vi "Test DMM-Readout.vi"() -> ()   [LabVIEW 2015, in "CS++DMM.lvlib"]
uses:
  CS++DMM.lvlib
  CSPP_Core/Classes/CS++BaseClasses/Factory/CS++Factory.lvclass
  CSPP_Core/Classes/CS++BaseClasses/Factory/CS++Factory.lvclass/CS++Factory.ctl
  CS++DMM.lvclass
  CSPP_Core/Actors/CS++DeviceActor/CS++DeviceActor.lvclass/CS++DeviceActor.ctl
  CSPP_Core/Actors/CS++DeviceActor/Read Resource Name.vi
  CSPP_Core/Actors/CS++DeviceActor/CS++DeviceActor.lvclass
  CSPP_Core/Actors/CS++BaseActor/CS++BaseActor.lvclass
panel:
  in  "CS++Object Names":string[](array[string])=["DMM3458A-GPIB0-21", "DMM3458A-GPIB0-22"]
  out "Last Time":timestamp format="%<%H:%M:%S%1u>T"
  in  "File Path Control":path=path "C:/User/Brand/LVP/STF/STF.ini"
  out "error out":errorcluster
  in  "Stop Button":bool
  out "Readings":dbl[](array[numeric])
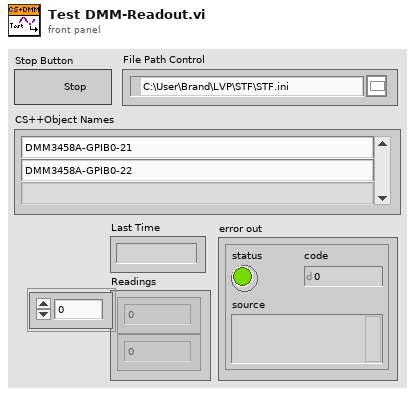
[diagram p1: front panel]
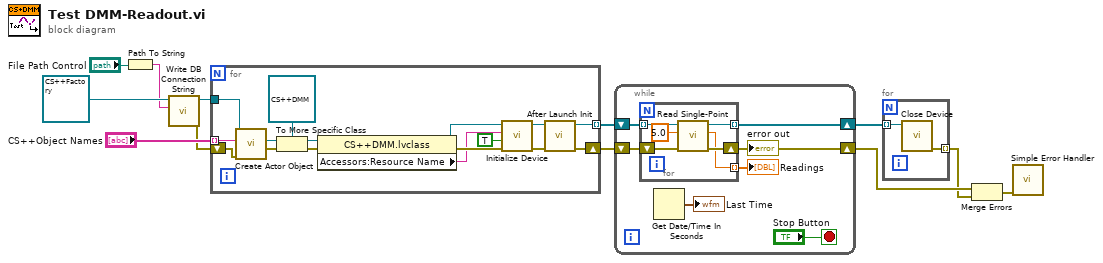
[diagram p0: block diagram]
diagram:
  n1 = Path To String(path="File Path Control") -> (string=w6:string)
  n2 = call "Write DB Connection String.vi"("DB Connection String"=w6, "CS++Factory in"=refnum<class "CS++Factory.lvclass"> refnum ("CS++BaseClasses.lvlib:CS++Factory.lvclass")) -> ("error out"=w1:errorcluster, "CS++Factory out"=w8:refnum<class "CS++Factory.lvclass">)  [unwired: 8 in]
  n3 = for {
    tunnel: w8 -> [w28]
    tunnel: "CS++Object Names" -> [w23] mode=indexing
    tunnel: [w16] -> w12 mode=indexing
    shift-right: [w14] -> w11
    shift-left: w1 -> [w13]
    n4 = call "Create Actor Object.vi"("error in (no error)"=w13, "Object Name"=w23, "CS++Factory in"=w28) -> ("error out"=w26:errorcluster, "CS++BaseActor"=w27:refnum<class "CS++BaseActor.lvclass">)  [unwired: 5 in, 2 out]
    n5 = To More Specific Class(target class=refnum<class "CS++DMM.lvclass"> refnum ("CS++DMM.lvlib:CS++DMM.lvclass"), reference=w27, error in=w26) -> (specific class reference=w24:refnum<class "CS++DMM.lvclass">, error out=w21:errorcluster)
    n6 = property class="CS++DMM.lvclass"(reference=w24, error in=w21) -> (reference out=w22:refnum<class "CS++DMM.lvclass">, error out=w20:errorcluster, "Accessors:Resource Name"=w19:string)
    n7 = call "Initialize Device.vi"("error in (no error)"=w20, "Reset (F)"=TRUE, "Resource Name"=w19, "CS++DeviceActor in"=w22) -> ("error out"=w15:errorcluster, "CS++DeviceActor out"=w17:refnum<class "CS++DMM.lvclass">)  [unwired: 6 in]
    n8 = call "After Launch Init.vi"("error in (no error)"=w15, "CS++BaseActor in"=w17) -> ("error out"=w14:errorcluster, "CS++BaseActor out"=w16:refnum<class "CS++DMM.lvclass">)  [unwired: 8 in]
  }
  n9 = while {
    shift-right: [w33] -> w5
    shift-left: w11 -> [w34]
    shift-right: [w32] -> w10
    shift-left: w12 -> [w35]
    stop <- "Stop Button" stop-if-true
    n10 = for {
      tunnel: w35 -> [w41] mode=indexing
      tunnel: [w38] -> w32 mode=indexing
      shift-right: [w39] -> w33
      shift-left: w34 -> [w40]
      tunnel: [w37] -> w31 mode=indexing
      n11 = call "Read Single-Point.vi"("error in (no error)"=w40, "maximum time (5s)"=dbl[unit] 5.0, "CS++DMM in"=w41) -> ("error out"=w39:errorcluster, "reading"=w37:dbl, "CS++DMM out"=w38:refnum<class "CS++DMM.lvclass">)  [unwired: 6 in]
    }
    "Readings" <- w31
    "error out" <- w33
    n12 = Get Date/Time In Seconds() -> (seconds since 1Jan1904=→"Last Time":timestamp)
  }
  n13 = for {
    tunnel: w10 -> [w43] mode=indexing
    tunnel: [w42] -> w4 mode=indexing
    n14 = call "Close Device.vi"("CS++DeviceActor in"=w43) -> ("error out"=w42:errorcluster)  [unwired: 9 in, 1 out]
  }
  n15 = Merge Errors(w5, w4) -> (w3:errorcluster)
  n16 = call <vilib>:"Simple Error Handler.vi"("error in (no error)"=w3) -> ()  [unwired: 4 in, 5 out]
